vi "DecodeData.vi"(8 "error in (no error)":errorcluster, 9 "Secret":string, 10 "Encoded Data":string, 11 "CryptoType":refnum<class "Crypto.AES.lvclass">) -> (0 "error out":errorcluster, 2 "Decoded Data":variant)   [LabVIEW 2016, in "Crypto.AES.lvclass"]
uses:
  Crypto.AES.lvclass
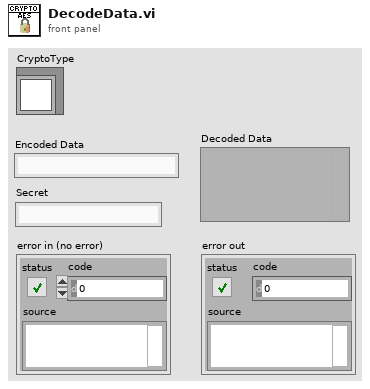
[diagram p1: front panel]
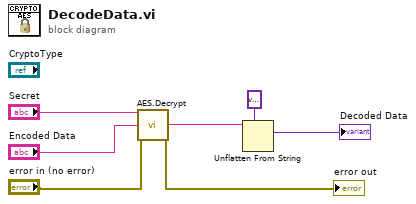
[diagram p0: block diagram]
diagram:
  n1 = call <vilib>:"AES.Decrypt.vi"("Password"="Secret", "EncryptedText"="Encoded Data", "error in"="error in (no error)") -> ("Plain Text"=w3:string, "error out"=→"error out":errorcluster)  [unwired: 11 in]
  n2 = Unflatten From String(type=variant, binary string=w3) -> (value=→"Decoded Data":variant)  [unwired: 3 in, 2 out]
